vi "escape and sum.vi"(11 "List in":dbl[](array[numeric])) -> (3 "List Out":dbl[](array[numeric]))   [LabVIEW 2023]
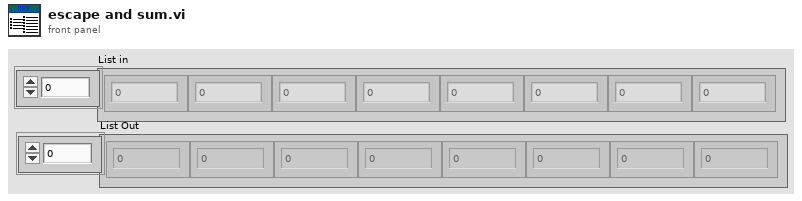
[diagram p1: front panel]
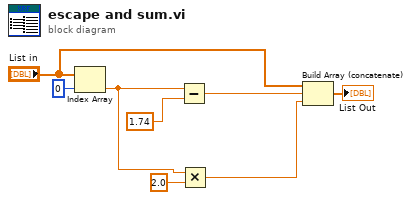
[diagram p0: block diagram]
diagram:
  n1 = Index Array(array="List in", index=0) -> (element=w5:dbl)
  n2 = Subtract(x=w5, y=1.74) -> (x-y=w3:dbl)
  n3 = Multiply(x=w5, y=2.0) -> (x*y=w4:dbl)
  n4 = Build Array (concatenate)("List in", w3, w4) -> (→"List Out":dbl[])
